vi "VacfPercentToI8.vi"(1 "vacf (0-100)":dbl) -> (0 "Accurus Ctrl Cluster":T1={"Stop Vacuum"=TRUE, "Vacuum Force"=0, "Max Limit [mmHg]"=600.0, "Slide in"=0, "Irrigation?"=TRUE})   [LabVIEW 2016]
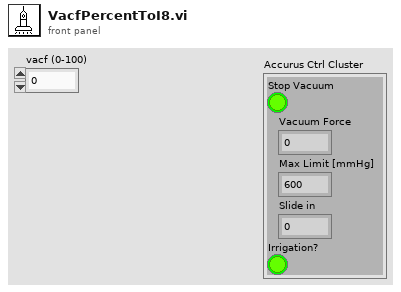
[diagram p1: front panel]
types:
  T1 = cluster{"Stop Vacuum":bool, "Vacuum Force":i8, "Max Limit [mmHg]":dbl, "Slide in":i8, "Irrigation?":bool}
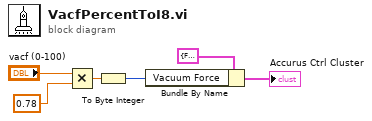
[diagram p0: block diagram]
diagram:
  n1 = Multiply(x="vacf (0-100)", y=0.78 ("x")) -> (x*y=w2:dbl)
  n2 = To Byte Integer(number=w2) -> (8bit integer=w3:i8)
  n3 = Bundle By Name(cluster=T1 {"Stop Vacuum"=FALSE, "Vacuum Force"=0, "Max Limit [mmHg]"=600.0, "Slide in"=0, "Irrigation?"=TRUE} ("Accurus Ctrl Cluster"), "Vacuum Force"=w3) -> (→"Accurus Ctrl Cluster":T1)
